vi "Prime Check.vi"() -> ()   [LabVIEW 2012]
panel:
  out "String":string
  in  "Numeric":dbl
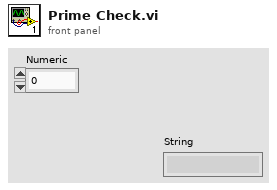
[diagram p1: front panel]
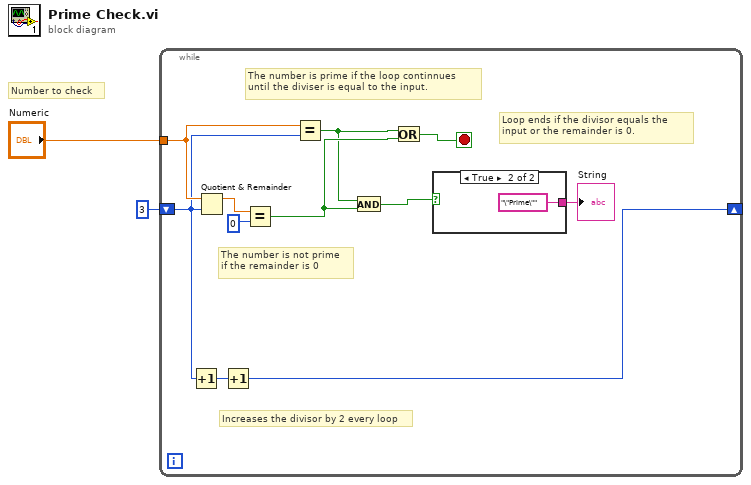
[diagram p0: block diagram]
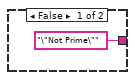
[diagram p2: hidden frame]
diagram:
  # "Number to check"
  n1 = while {
    tunnel: "Numeric" -> [w13]
    shift-right: [w8] -> _
    shift-left: 3 -> [w7]
    stop <- w10 stop-if-true
    # "Loop ends if the divisor equals the input or the remainder is 0."
    # "The number is prime if the loop continnues \nuntil the diviser is equal to the input."
    # "Increases the divisor by 2 every loop"
    # "The number is not prime\nif the remainder is 0"
    n2 = Increment(x=w7) -> (x+1=w9:i32)
    n3 = Quotient & Remainder(x=w13, y=w7) -> (x-y*floor(x/y)=w12:dbl)  [unwired: 1 out]
    n4 = Increment(x=w9) -> (x+1=w8:i32)
    n5 = Equal?(x=w12, y=0) -> (x = y?=w4:bool)
    n6 = Equal?(x=w13, y=w7) -> (x = y?=w3:bool)
    n7 = And(x=w3, y=w4) -> (x .and. y?=w6:bool)
    n8 = Or(x=w3, y=w4) -> (x .or. y?=w10:bool)
    n9 = case shown="True" w6 {
      tunnel: ["\"Not Prime\"" "\"Prime\""] -> w5
      frame False {
      }
      frame True {
      }
    }
    "String" <- w5
  }
